vi "PC Benchmarking UI.vi"() -> ()   [LabVIEW 2014]
panel:
  out "Input Time":dbl(graph)
  out "Output Time":dbl
  out "Process Time":dbl
  out "Loop Start Time":dbl
  in  "Boolean In":bool
  in  "I32 In":i32
  in  "Single In":sgl
  in  "Double In":dbl
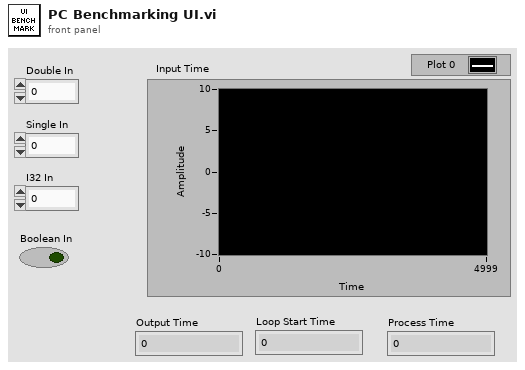
[diagram p1: front panel]
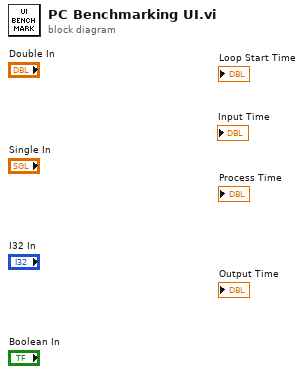
[diagram p0: block diagram]
diagram:
